vi "Security System Demo.vi"() -> ()   [LabVIEW 2020]
uses:
  Security System/Security Level.ctl
  Door Alarm/Door Alarm.lvclass
  D:/LabVIEW/LabVIEW codes/solutions_and_repetitions/Channel_pattern/Security System/Security System.lvclass
  Motions Detectors/Motion Detectors.lvclass
  Threat Deterent/Threat Deterents.lvclass
  Security System/Security System.lvclass
panel:
  in  "stop":bool
  out "Last Action Performed":string
  in  "Security Level":T1
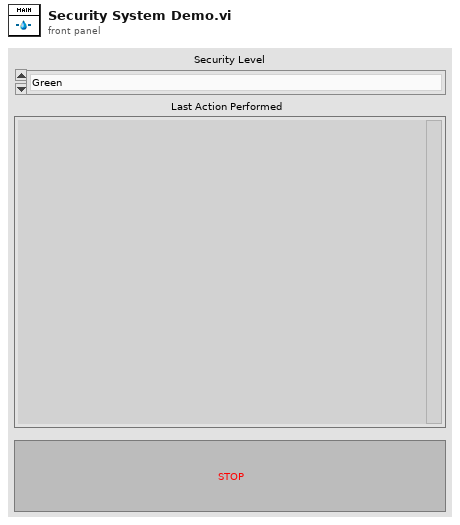
[diagram p1: front panel]
types:
  T1 = typedef "Security System.lvclass/Security Level.ctl" = enum16{"Green", "Yellow", "Orange", "Red"}
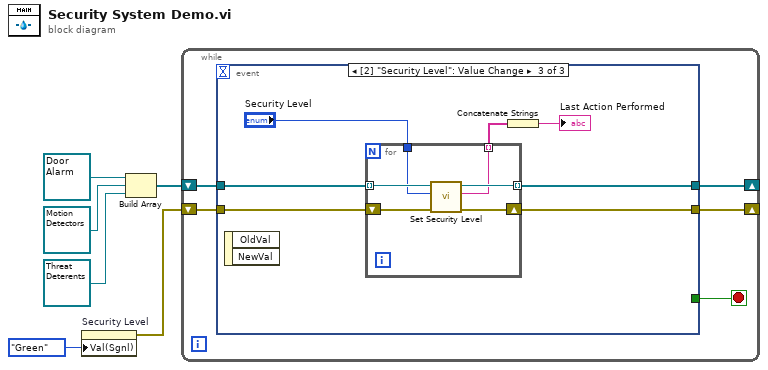
[diagram p0: block diagram]
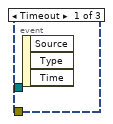
[diagram p2: hidden frame]
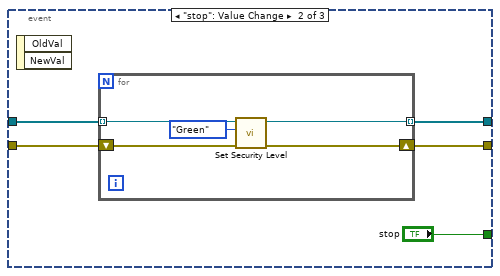
[diagram p3: hidden frame]
diagram:
  n1 = property on="Security Level" class="Enum (strict)"("Val(Sgnl)"=Security_Level."Green" ("Value (Signaling)")) -> (error out=w1:errorcluster)  [unwired: 2 in, 1 out]
  n2 = Build Array(refnum<class "Door Alarm.lvclass"> refnum ("Door Alarm.lvclass"), refnum<class "Motion Detectors.lvclass"> refnum ("Motion Detectors.lvclass"), refnum<class "Threat Deterents.lvclass"> refnum ("Threat Deterents.lvclass")) -> (w3:refnum<class "Security System.lvclass">[])
  n3 = while {
    shift-right: [w8] -> _
    shift-left: w3 -> [w11]
    shift-right: [w7] -> _
    shift-left: w1 -> [w10]
    stop <- w9 stop-if-true
    n4 = event shown="[2] \"Security Level\": Value Change" {
      selector: _ -> [_ _ _]
      dyn-events: _ -> [_ _ _]
      timeout: _ -> [_ _ _]
      tunnel: w11 -> [_ w15 w28]
      tunnel: w10 -> [_ w14 w27]
      tunnel: [_ "stop" _] -> w9
      tunnel: [_ w13 w25] -> w8
      tunnel: [_ w12 w26] -> w7
      event Timeout {
        n5 = event-data() -> ()  [unwired: 1 in, 3 out]
      }
      event "stop": Value Change {
        n6 = event-data() -> ()  [unwired: 1 in, 2 out]
        n7 = for {
          tunnel: w15 -> [w20] mode=indexing
          shift-right: [w18] -> w12
          shift-left: w14 -> [w21]
          tunnel: [w19] -> w13 mode=indexing
          n8 = call "Set Security Level.vi"("error in (no error)"=w21, "New Level"=Security_Level."Green", "Security System in"=w20) -> ("error out"=w18:errorcluster, "Security System out"=w19:refnum<class "Security System.lvclass">)  [unwired: 6 in, 1 out]
        }
      }
      event Value Change {
        n9 = event-data() -> ()  [unwired: 1 in, 2 out]
        n10 = for {
          tunnel: w28 -> [w34] mode=indexing
          shift-right: [w32] -> w26
          shift-left: w27 -> [w33]
          tunnel: [w31] -> w25 mode=indexing
          tunnel: "Security Level" -> [w30]
          tunnel: [w29] -> w23 mode=indexing
          n11 = call "Set Security Level.vi"("error in (no error)"=w33, "New Level"=w30, "Security System in"=w34) -> ("error out"=w32:errorcluster, "Last Action Performed"=w29:string, "Security System out"=w31:refnum<class "Security System.lvclass">)  [unwired: 6 in]
        }
        n12 = Concatenate Strings(w23) -> (→"Last Action Performed":string)
      }
    }
  }
